vi "AddFilter.vi"(8 "Bottom":i16, 9 "Right":i16, 10 "Output 1":u8[][](array[numeric]), 11 "Filters":T1(ring)) -> (3 "Filtered X":dbl[][](array[numeric]))   [LabVIEW 2016]
uses:
  <vilib>/Analysis/3filter.llb/Equi-Ripple LowPass (DBL).vi
  <vilib>/Analysis/3filter.llb/Equi-Ripple HighPass (DBL).vi
  <vilib>/Analysis/3filter.llb/Equi-Ripple BandPass (DBL).vi
  <vilib>/Analysis/3filter.llb/Equi-Ripple BandStop (DBL).vi
  <vilib>/Analysis/3filter.llb/Butterworth Filter (DBL).vi
  <vilib>/Analysis/NI_AALBase.lvlib
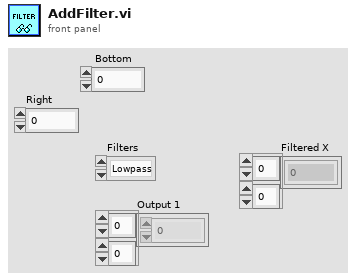
[diagram p1: front panel]
types:
  T1 = enum32{"Lowpass ", "Highpass", "Band pass", "Band Stop", "Butter Worth ", "No filter"}
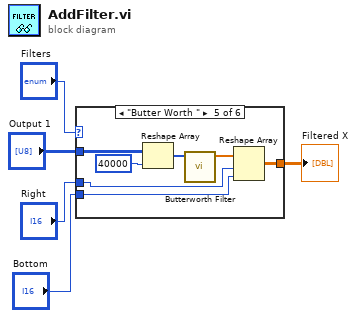
[diagram p0: block diagram]
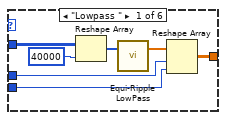
[diagram p2: hidden frame]
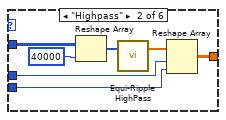
[diagram p3: hidden frame]
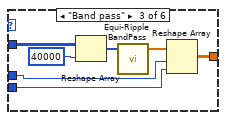
[diagram p4: hidden frame]
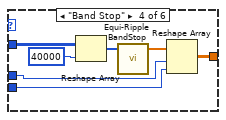
[diagram p5: hidden frame]
diagram:
  n1 = case shown="\"Butter Worth \"" "Filters" {
    tunnel: "Output 1" -> [w9 w18 w25 w32 w39 w41]
    tunnel: [w8 w15 w22 w31 w36 w41] -> w3
    tunnel: "Right" -> [w7 w14 w21 w28 w35 _]
    tunnel: "Bottom" -> [w6 w13 w20 w27 w34 _]
    frame "Lowpass " {
      n2 = Reshape Array(w9, 40000 ("dimension size")) -> (w11:u8[])
      n3 = call-poly <vilib>:"Equi-Ripple LowPass.vi"("X"=w11) -> ("Filtered X"=w10:dbl[])  [unwired: 5 in, 1 out]
      n4 = Reshape Array(w10, w7, w6) -> (w8:dbl[][])
    }
    frame "Highpass" {
      n5 = Reshape Array(w18, 40000 ("dimension size")) -> (w17:u8[])
      n6 = call-poly <vilib>:"Equi-Ripple HighPass.vi"("X"=w17) -> ("Filtered X"=w16:dbl[])  [unwired: 5 in, 1 out]
      n7 = Reshape Array(w16, w14, w13) -> (w15:dbl[][])
    }
    frame "Band pass" {
      n8 = Reshape Array(w25, 40000 ("dimension size")) -> (w24:u8[])
      n9 = call-poly <vilib>:"Equi-Ripple BandPass.vi"("X"=w24) -> ("Filtered X"=w23:dbl[])  [unwired: 7 in, 1 out]
      n10 = Reshape Array(w23, w21, w20) -> (w22:dbl[][])
    }
    frame "Band Stop" {
      n11 = Reshape Array(w32, 40000 ("dimension size")) -> (w30:u8[])
      n12 = call-poly <vilib>:"Equi-Ripple BandStop.vi"("X"=w30) -> ("Filtered X"=w29:dbl[])  [unwired: 7 in, 1 out]
      n13 = Reshape Array(w29, w28, w27) -> (w31:dbl[][])
    }
    frame "Butter Worth " {
      n14 = Reshape Array(w39, 40000 ("dimension size")) -> (w38:u8[])
      n15 = call-poly <vilib>:"Butterworth Filter.vi"("X"=w38) -> ("Filtered X"=w37:dbl[])  [unwired: 7 in, 1 out]
      n16 = Reshape Array(w37, w35, w34) -> (w36:dbl[][])
    }
    frame "No filter", Default {
    }
  }
  "Filtered X" <- w3
